vi "stopMotion.vi"(8 "error in (no error)":errorcluster, 10 "model":refnum<class "Model.lvclass">, 11 "TestingState in":refnum<class "TestingState.lvclass">) -> (0 "error out":errorcluster, 2 "model 2":refnum<class "Model.lvclass">, 3 "TestingState out":refnum<class "TestingState.lvclass">)   [LabVIEW 2015]
uses:
  Model/Model/Model.lvclass
  TestingState.lvclass
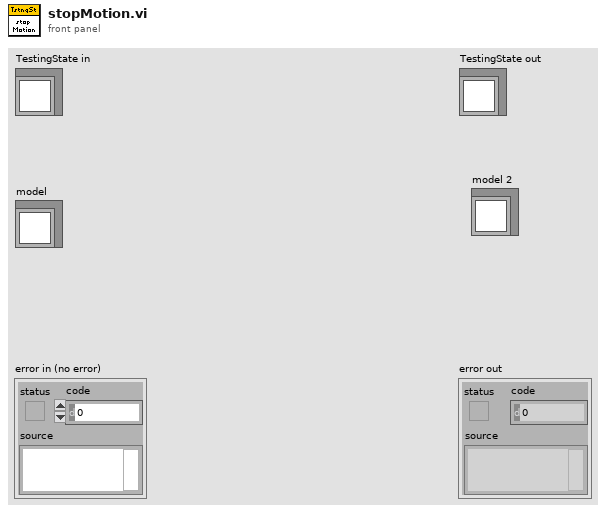
[diagram p1: front panel]
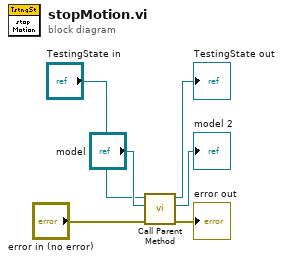
[diagram p0: block diagram]
diagram:
  n1 = call-parent "Call Parent Method"("error in (no error)"="error in (no error)", "model"="model", "State in"="TestingState in") -> ("error out"=→"error out":errorcluster, "model 2"=→"model 2":refnum<class "Model.lvclass">, "State out"=→"TestingState out":refnum<class "TestingState.lvclass">)  [unwired: 6 in]
